vi "CreateNewWizard_IncludeItem.vi"(11 "Wizard":T1) -> (3 "Include me":bool)   [LabVIEW 2020, in "Add Actor Interface.lvlib"]
uses:
  Add Actor Interface.lvlib
  MessageMakerProvider/_Message Maker/Message Maker.lvlib
  <resource>/Framework/Providers/API/ItemRef.ctl
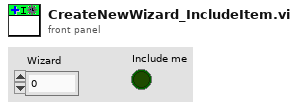
[diagram p1: front panel]
types:
  T1 = typedef "ItemRef.ctl" = u64
  T2 = typedef "mxLvNIIM.ctl" = cluster{"Item URL":string, "Item ID":string, "Item Index":i32, "Specific Type":string}
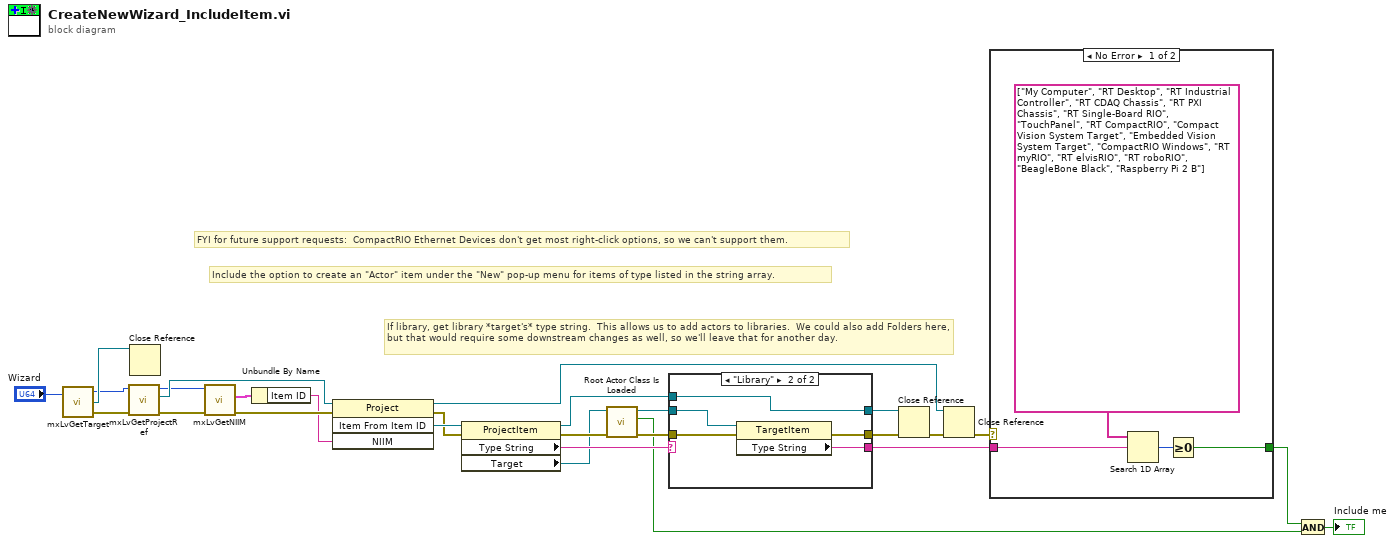
[diagram p0: block diagram]
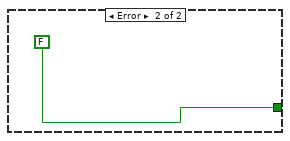
[diagram p3: hidden frame]
diagram:
  # "FYI for future support requests:  CompactRIO Ethernet Devices don't get most right-click options, so we can't support them."
  # "If library, get library *target's* type string.  This allows us to add actors to libraries.  We could also add Folders here, but that would require some downstream changes as well, so we'll leave that for another day."
  # "Include the option to create an \"Actor\" item under the \"New\" pop-up menu for items of type listed in the string array."
  n1 = call <resource>:"mxLvGetTarget.vi"("Item"="Wizard") -> ("Item"=w20:T1, "Target"=w22:refnum<vi>, "error out"=w21:errorcluster)  [unwired: 1 in]
  n2 = call <resource>:"mxLvGetProjectRef.vi"("error in"=w21, "Item"=w20) -> ("error out"=w27:errorcluster, "Project Refnum"=w23:refnum<vi>, "Item"=w18:T1)  [unwired: 7 in]
  n3 = Close Reference(reference=w22) -> ()  [unwired: 1 in, 1 out]
  n4 = call <resource>:"mxLvGetNIIM.vi"("error in"=w27, "Item"=w18) -> ("error out"=w25:errorcluster, "NIIM"=w24:T2)  [unwired: 7 in, 1 out]
  n5 = Unbundle By Name(w24) -> ("Item ID"=w8:string)
  n6 = invoke class="Project" method="Item From Item ID"(reference=w23, error in=w25, "NIIM"=w8) -> (reference out=w11:refnum<vi>, error out=w16:errorcluster, "GetItemFromNIIM"=w26:refnum<vi>)  [unwired: 1 in, 1 out]
  n7 = property class="ProjectItem"(reference=w26, error in=w16) -> (reference out=w17:refnum<vi>, error out=w7:errorcluster, "Type String"=w10:string, "Target"=w5:refnum<vi>)
  n8 = call "Root Actor Class Is Loaded.vi"("error in (no error)"=w7, "TargetItem in"=w5) -> ("error out"=w6:errorcluster, "is Actor.lvclass loaded already?"=w3:bool, "TargetItem out"=w4:refnum<vi>)  [unwired: 7 in]
  n9 = case shown="\"Library\"" w10 {
    selector: w10 -> [w28 _]
    tunnel: w6 -> [w29 w31]
    tunnel: w17 -> [w30 w32]
    tunnel: [w28 w35] -> w9
    tunnel: [w29 w34] -> w15
    tunnel: [w30 w32] -> w14
    tunnel: w4 -> [_ w33]
    frame Default {
    }
    frame "Library" {
      n10 = property class="TargetItem"(reference=w33, error in=w31) -> (error out=w34:errorcluster, "Type String"=w35:string)  [unwired: 1 out]
    }
  }
  n11 = Close Reference(reference=w14, error in (no error)=w15) -> (error out=w13:errorcluster)
  n12 = Close Reference(reference=w11, error in (no error)=w13) -> (error out=w12:errorcluster)
  n13 = case shown="No Error" w12 {
    tunnel: w9 -> [w39 _]
    tunnel: [w37 FALSE] -> w2
    frame No Error {
      n14 = Search 1D Array(1D array=string[] ["My Computer", "RT Desktop", "RT Industrial Controller", "RT CDAQ Chassis", "RT PXI Chassis", "RT Single-Board RIO", "TouchPanel", "RT CompactRIO", "Compact Vision System Target", "Embedded Vision System Target", "CompactRIO Windows", "RT myRIO", "RT elvisRIO", "RT roboRIO", "BeagleBone Black", "Raspberry Pi 2 B"] ("Array"), element=w39) -> (index of element=w38:i32)  [unwired: 1 in]
      n15 = Greater Or Equal To 0?(x=w38) -> (x >= 0?=w37:bool)
    }
    frame Error {
    }
  }
  n16 = And(x=w2, y=w3) -> (x .and. y?=→"Include me":bool)
